vi "timerstamp.vi"() -> ()   [LabVIEW 2024]
panel:
  out "Waveform Chart":dbl(graph)
  out "output waveform":waveform(dbl)
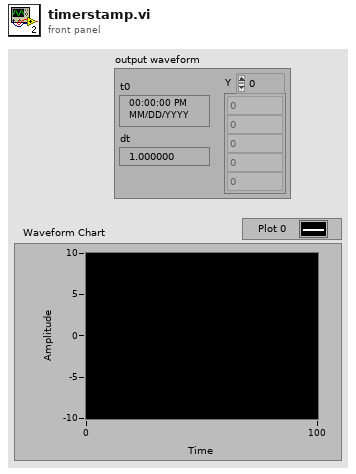
[diagram p1: front panel]
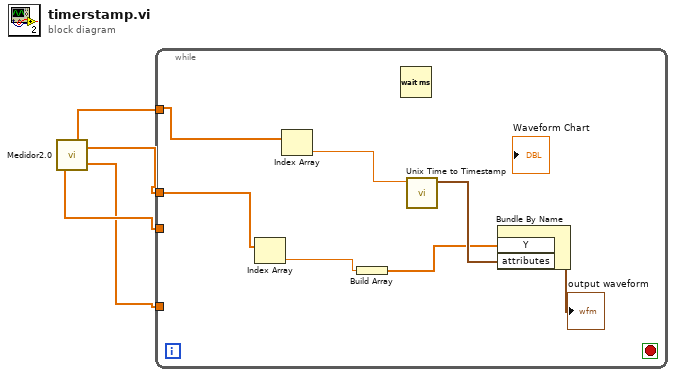
[diagram p0: block diagram]
diagram:
  n1 = call "Medidor2.0.vi"() -> ("Potencia ativa C"=w1:dbl[], "Potencia ativa A"=w3:dbl[], "Potencia ativa B"=w2:dbl[], "TimeStamp"=w4:dbl[])
  n2 = while {
    tunnel: w4 -> [w11]
    tunnel: w3 -> [w10]
    tunnel: w2 -> [_]
    tunnel: w1 -> [_]
    stop <- _ stop-if-true
    n3 = Index Array(array=w10) -> (element=w6:dbl)  [unwired: 1 in]
    n4 = Index Array(array=w11) -> (element=w8:dbl)  [unwired: 1 in]
    n5 = Build Array(w6) -> (w5:dbl[])
    n6 = Wait (ms)() -> ()  [unwired: 1 in, 1 out]
    n7 = call <vilib>:"Unix Time to Timestamp.vi"("Unix Time (s)"=w8) -> ("Timestamp"=w7:timestamp)  [unwired: 9 in, 1 out]
    n8 = Bundle By Name("Y"=w5, "attributes"=w7) -> (→"output waveform":waveform(dbl))  [unwired: 1 in]
  }
